vi "ReadAllCtlRefs_Core.vi"(8 "error in (no error)":errorcluster, 11 "ctlRef_Maps in":refnum<class "ctlRef_Maps.lvclass">) -> (0 "error out":errorcluster, 1 "Values":refnum<vi>[](array[refnum]), 2 "Names":string[](array[string]), 3 "ctlRef_Maps out":refnum<class "ctlRef_Maps.lvclass">)   [LabVIEW 2020, in "CtlReferences.lvlib" / "ctlRef_Maps.lvclass"]
uses:
  ctlRef_Maps.lvclass
  ctlRef_Maps.lvclass/ctlRef_Maps.ctl
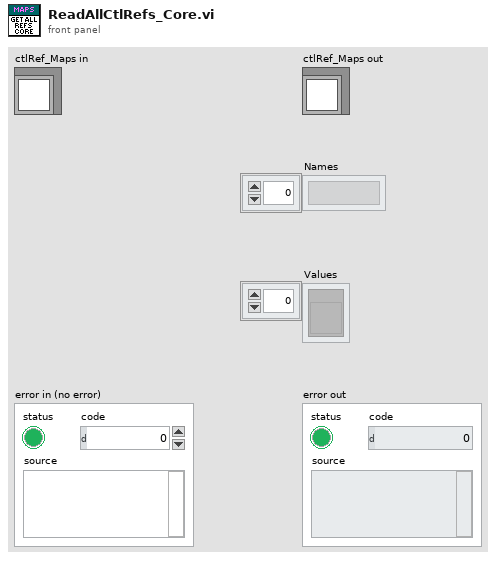
[diagram p1: front panel]
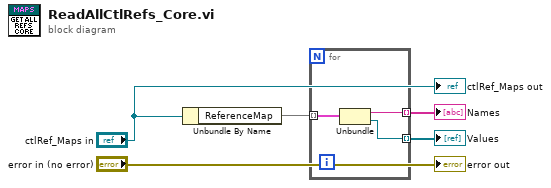
[diagram p0: block diagram]
diagram:
  n1 = Unbundle By Name("ctlRef_Maps in") -> ("ReferenceMap"=w3:map{string, refnum<vi>})
  n2 = for {
    tunnel: w3 -> [w8] mode=indexing
    tunnel: [w7] -> w2 mode=indexing
    tunnel: [w6] -> w1 mode=indexing
    n3 = Unbundle(w8) -> ("Name"=w7:string, "Reference"=w6:refnum<vi>)
  }
  "Values" <- w1
  "Names" <- w2
  "ctlRef_Maps out" <- "ctlRef_Maps in"
  "error out" <- "error in (no error)"
